vi "Write Channel.vi"(8 "error in (no error)":errorcluster, 10 "Channel":i32, 11 "Set Output Value Msg in":refnum<class "Set Output Value Msg.lvclass">) -> (0 "error out":errorcluster, 3 "Set Output Value Msg out":refnum<class "Set Output Value Msg.lvclass">)   [LabVIEW 2016, in "BNT_DAQmx.lvlib" / "Set Output Value Msg.lvclass"]
uses:
  Set Output Value Msg.lvclass
  Set Output Value Msg.lvclass/Set Output Value Msg.ctl
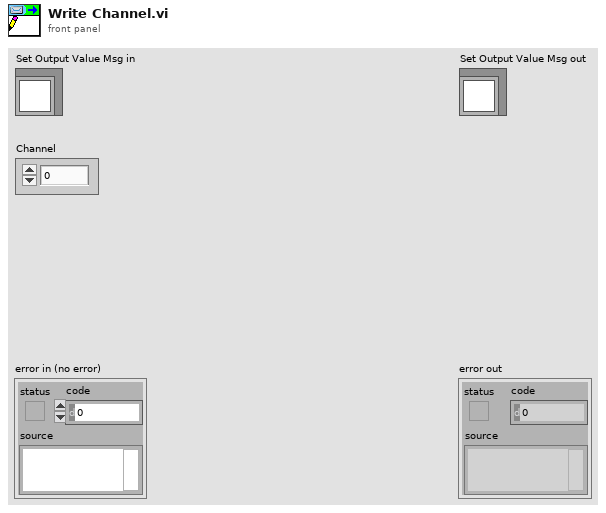
[diagram p1: front panel]
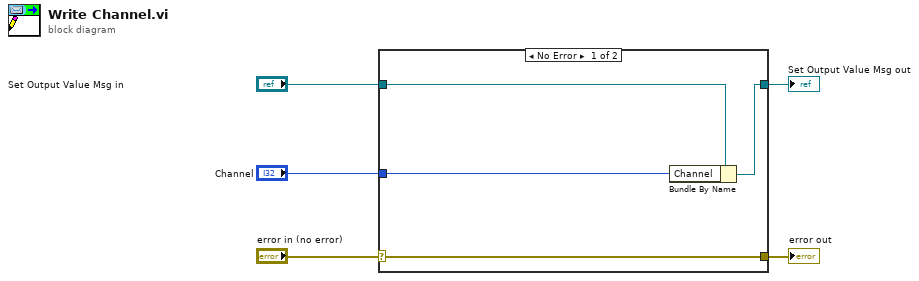
[diagram p0: block diagram]
diagram:
  n1 = case shown="No Error" "error in (no error)" {
    selector: "error in (no error)" -> [w9 w10]
    tunnel: [w9 w10] -> w4
    tunnel: [w7 w11] -> w2
    tunnel: "Set Output Value Msg in" -> [w8 w11]
    tunnel: "Channel" -> [w6 _]
    frame No Error {
      n2 = Bundle By Name(cluster=w8, "Channel"=w6) -> (w7:refnum<class "Set Output Value Msg.lvclass">)
    }
    frame Error {
    }
  }
  "error out" <- w4
  "Set Output Value Msg out" <- w2
